vi "Memory.Array.Allocate.vi"(7 "allocation limit (2^31: 2GiB)":i64=2147483647 format="%08x bytes", 8 "error in (no error)":errorcluster, 9 "number of elements":u64, 10 "size of element":i64 format="%d bytes", 11 "Array in":refnum<class "Memory.Array.Void.lvclass">) -> (0 "error out":errorcluster, 2 "allocated size":i64 format="%d bytes", 3 "Array out":refnum<class "Memory.Array.Void.lvclass">)   [LabVIEW 2016, in "LabVIEW Memory Manager.lvlib" / "Memory.Array.Void.lvclass"]
uses:
  Memory.Array.Void.lvclass
  Pointer/Pointer.Void/Memory.Pointer.Void.lvclass/Memory.Pointer.Void.ctl
  Memory.Array.Void.lvclass/Memory.Array.Void.ctl
  Pointer/Pointer.Void/Methods/Memory.Pointer.Allocate.vi
  Pointer/Pointer.Void/Methods/Memory.Pointer.Set Address.vi
  Pointer/Pointer.Void/Methods/Memory.Pointer.Set Size.vi
  Pointer/Pointer.Void/Memory.Pointer.Void.lvclass
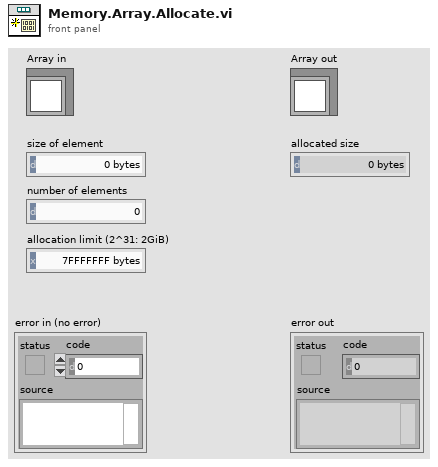
[diagram p1: front panel]
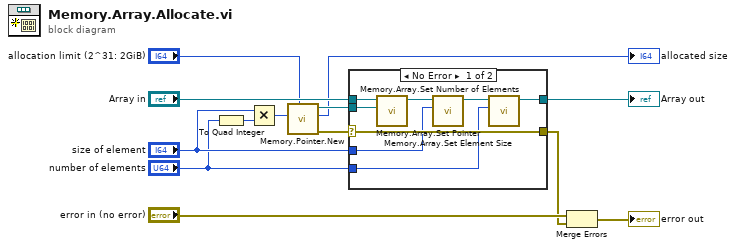
[diagram p0: block diagram]
diagram:
  n1 = To Quad Integer(1:"number of elements") -> (0:w8:i64)
  n2 = Multiply(x="size of element", y=w8) -> (x*y=w7:i64)
  n3 = call "Memory.Pointer.New.vi"("allocation limit (2^31: 2GiB)"="allocation limit (2^31: 2GiB)", "size"=w7) -> ("error out"=w12:errorcluster, "allocated size"=→"allocated size":u64, "Pointer out"=w13:refnum<class "Memory.Pointer.Void.lvclass">)  [unwired: 7 in]
  n4 = case shown="No Error" w12 {
    selector: w12 -> [w20 w22]
    tunnel: w13 -> [w19 _]
    tunnel: "Array in" -> [w21 w23]
    tunnel: [w16 w23] -> w3
    tunnel: [w20 w22] -> w9
    tunnel: "size of element" -> [w14 _]
    tunnel: "number of elements" -> [w15 _]
    frame No Error {
      n5 = call "Memory.Array.Set Pointer.vi"("Pointer"=w19, "Array in"=w21) -> ("Array out"=w18:refnum<class "Memory.Array.Void.lvclass">)  [unwired: 8 in, 1 out]
      n6 = call "Memory.Array.Set Element Size.vi"("size of element"=w14, "Memory.Array in"=w18) -> ("Memory.Array out"=w17:refnum<class "Memory.Array.Void.lvclass">)  [unwired: 8 in, 1 out]
      n7 = call "Memory.Array.Set Number of Elements.vi"("number of elements"=w15, "Memory.Array in"=w17) -> ("Memory.Array out"=w16:refnum<class "Memory.Array.Void.lvclass">)  [unwired: 8 in, 1 out]
    }
    frame Error {
    }
  }
  "Array out" <- w3
  n8 = Merge Errors("error in (no error)", w9) -> (→"error out":errorcluster)
